vi "Scorer Done.vi"(8 "error in (no error)":errorcluster, 10 "Scorer":refnum<class "Scorer.lvclass">, 11 "SOL-Server in":refnum<class "SOL-Server.lvclass">) -> (0 "error out":errorcluster, 3 "SOL-Server out":refnum<class "SOL-Server.lvclass">)   [LabVIEW 2020, in "Summer of LabVIEW.lvlib" / "SOL-Server.lvclass"]
uses:
  SOL-Server.lvclass
  Scorer/Scorer.lvclass
  SOL-Server.lvclass/SOL-Server.ctl
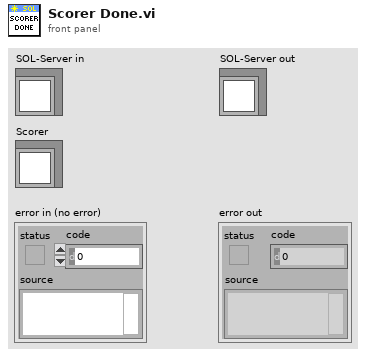
[diagram p1: front panel]
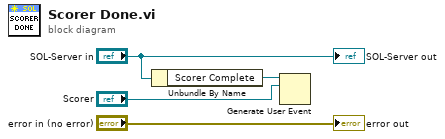
[diagram p0: block diagram]
diagram:
  n1 = Unbundle By Name("SOL-Server in") -> ("Scorer Complete"=w2:refnum<user-event>)
  n2 = Generate User Event(user event=w2, event data cluster="Scorer") -> ()  [unwired: 2 in, 2 out]
  "error out" <- "error in (no error)"
  "SOL-Server out" <- "SOL-Server in"
